vi "VI Tree - dictionary__ogtk.vi"   [LabVIEW 2018]
uses:
  <userlib>/_OpenG.lib/dictionary/dictionary.llb/Dictionary Key Value Pair Cluster__ogtk.ctl
panel:
  # "Dictionary VI Tree"
  # "Dictionary - VI Tree\n\nA VI that contains all of the Dictionary VIs\n\nPlease visit http://www.OpenG.org to learn about the\nOpen Source LabVIEW software movement.\n\nNOTICE -- YOU MUST LEAVE THIS NOTICE IN PLACE.  PER THE TERMS OF THE LICENSE BELOW, YOU MAY SUBLICENSE THIS SOFTWARE \nIN ANY WAY THAT DOES NOT CONFLICT WITH THIS LICENSE.\n\n### BSD License (http://www.opensource.org/licenses/bsd-license.php) Begin ###\n \nCopyright (c) 2005, Jim Kring <jim@jimkring.com>\n\nAll rights reserved.\n\nRedistribution and use in source and binary forms, with or without modification, are permitted provided that the following conditions are met:\n\n    * Redistributions of source code must retain the above copyright notice, this list of conditions and the following disclaimer.\n    * Redistributions in binary form must reproduce the above copyright notice, this list of conditions and the following disclaimer in the \n       documentation and/or other materials provided with the distribution.\n    * Neither the name of SciWare, James Kring, Inc., nor the names of its contributors may be used to endorse or promote products derived \n       from this software without specific prior written permission.\n\nTHIS SOFTWARE IS PROVIDED BY THE COPYRIGHT HOLDERS AND CONTRIBUTORS \"AS IS\" AND ANY EXPRESS OR IMPLIED WARRANTIES, \nINCLUDING, BUT NOT LIMITED TO, THE IMPLIED WARRANTIES OF MERCHANTABILITY AND FITNESS FOR A PARTICULAR PURPOSE ARE \nDISCLAIMED. IN NO EVENT SHALL THE COPYRIGHT OWNER OR CONTRIBUTORS BE LIABLE FOR ANY DIRECT, INDIRECT, INCIDENTAL,\n SPECIAL, EXEMPLARY, OR CONSEQUENTIAL DAMAGES (INCLUDING, BUT NOT LIMITED TO, PROCUREMENT OF SUBSTITUTE GOODS OR \nSERVICES; LOSS OF USE, DATA, OR PROFITS; OR BUSINESS INTERRUPTION) HOWEVER CAUSED AND ON ANY THEORY OF LIABILITY, \nWHETHER IN CONTRACT, STRICT LIABILITY, OR TORT (INCLUDING NEGLIGENCE OR OTHERWISE) ARISING IN ANY WAY OUT OF THE USE \nOF THIS SOFTWARE, EVEN IF ADVISED OF THE POSSIBILITY OF SUCH DAMAGE.\n\n### BSD License End ###"
types:
  T1 = typedef "Dictionary Key Value Pair Cluster__ogtk.ctl" = cluster{"key":variant, "value":variant}
  T2 = typedef "Dictionary Object RefNum__ogtk.ctl" = refnum<k1>
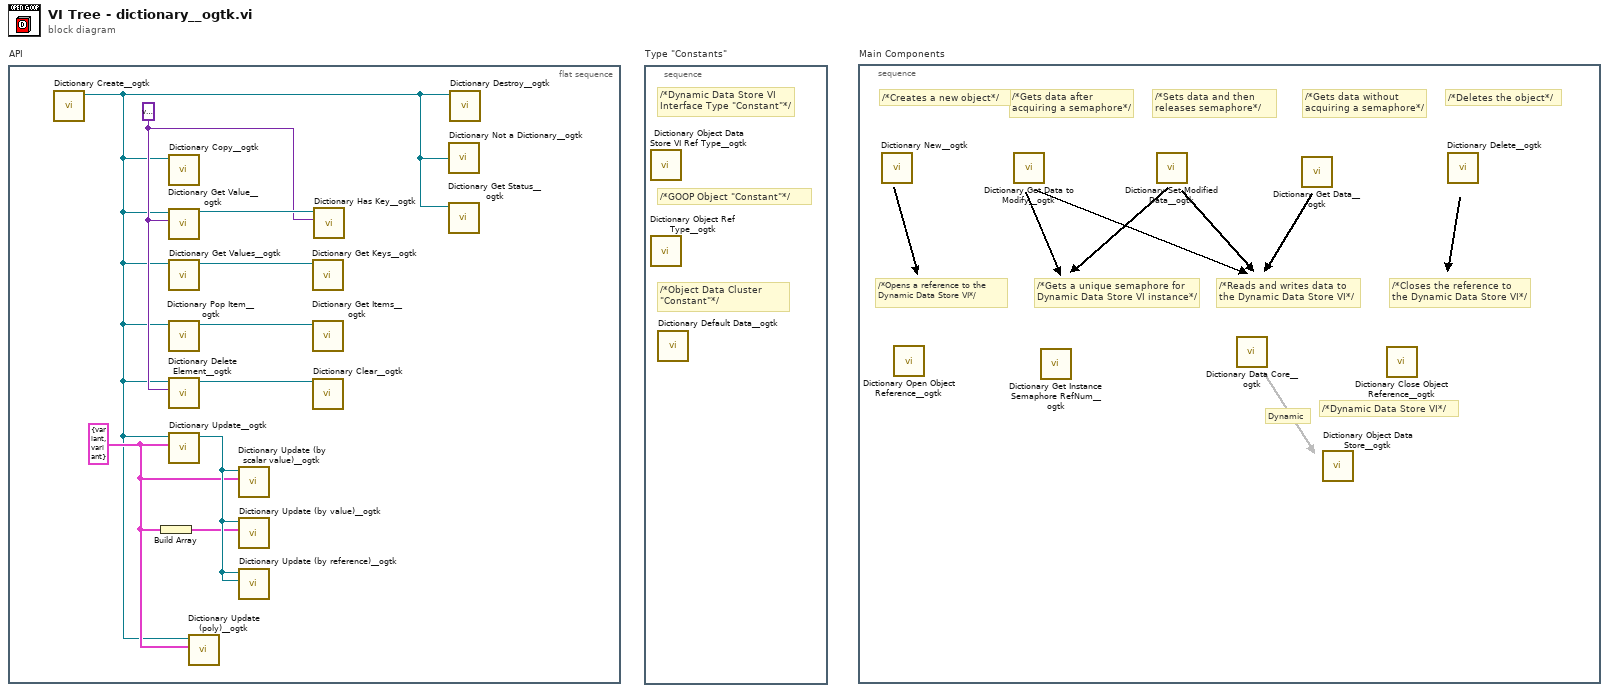
[diagram p0: block diagram]
diagram:
  n1 = flat-sequence "API" {
    frame #0 {
      w2 = T1 {"key"=variant, "value"=variant} ("key-value")
      w3 = variant ("key")
      n2 = call <userlib>:"Dictionary Create__ogtk.vi"() -> ("dictionary out"=w1:T2)  [unwired: 10 in, 1 out]
      n3 = Build Array(w2) -> (w4:T1[])
      n4 = call <userlib>:"Dictionary Copy__ogtk.vi"("dictionary"=w1) -> ()  [unwired: 8 in, 3 out]
      n5 = call <userlib>:"Dictionary Get Value__ogtk.vi"("key"=w3, "dictionary"=w1) -> ("dictionary out"=w5:T2)  [unwired: 6 in, 3 out]
      n6 = call <userlib>:"Dictionary Get Values__ogtk.vi"("dictionary"=w1) -> ("dictionary out"=w9:T2)  [unwired: 8 in, 2 out]
      n7 = call <userlib>:"Dictionary Pop Item__ogtk.vi"("dictionary"=w1) -> ("dictionary out"=w7:T2)  [unwired: 8 in, 2 out]
      n8 = call <userlib>:"Dictionary Delete Element__ogtk.vi"("key"=w3, "dictionary"=w1) -> ("dictionary out"=w6:T2)  [unwired: 8 in, 1 out]
      n9 = call-poly <userlib>:"Dictionary Update__ogtk.vi"("key-value"=w2, "dictionary"=w1) -> ("dictionary out"=w8:T2)  [unwired: 7 in, 2 out]
      n10 = call-poly <userlib>:"Dictionary Update (poly)__ogtk.vi"("key-value"=w2, "dictionary"=w1) -> ()  [unwired: 7 in, 3 out]
      n11 = call <userlib>:"Dictionary Update (by scalar value)__ogtk.vi"("key-value"=w2, "dictionary"=w8) -> ()  [unwired: 7 in, 3 out]
      n12 = call <userlib>:"Dictionary Update (by value)__ogtk.vi"("dictionary with updates"=w4, "dictionary"=w8) -> ()  [unwired: 7 in, 3 out]
      n13 = call <userlib>:"Dictionary Update (by reference)__ogtk.vi"("dictionary with updates"=w8, "dictionary"=w8) -> ()  [unwired: 7 in, 3 out]
      n14 = call <userlib>:"Dictionary Get Keys__ogtk.vi"("dictionary"=w9) -> ()  [unwired: 8 in, 3 out]
      n15 = call <userlib>:"Dictionary Get Items__ogtk.vi"("dictionary"=w7) -> ()  [unwired: 8 in, 3 out]
      n16 = call <userlib>:"Dictionary Clear__ogtk.vi"("dictionary"=w6) -> ()  [unwired: 9 in, 2 out]
      n17 = call <userlib>:"Dictionary Has Key__ogtk.vi"("key"=w3, "dictionary"=w5) -> ()  [unwired: 7 in, 3 out]
      n18 = call <userlib>:"Dictionary Not a Dictionary__ogtk.vi"("dictionary"=w1) -> ()  [unwired: 1 out]
      n19 = call <userlib>:"Dictionary Get Status__ogtk.vi"("dictionary"=w1) -> ()  [unwired: 8 in, 3 out]
      n20 = call <userlib>:"Dictionary Destroy__ogtk.vi"("dictionary"=w1) -> ()  [unwired: 10 in, 1 out]
    }
  }
  n21 = stacked-sequence "Type \"Constants\"" {
    frame #0 {
      # "/*Dynamic Data Store VI Interface Type \"Constant\"*/"
      # "/*GOOP Object \"Constant\"*/"
      # "/*Object Data Cluster \"Constant\"*/"
      n22 = call <userlib>:"Dictionary Object Data Store VI Ref Type__ogtk.vi"() -> ()  [unwired: 5 in, 1 out]
      n23 = call <userlib>:"Dictionary Object Ref Type__ogtk.vi"() -> ()  [unwired: 5 in, 1 out]
      n24 = call <userlib>:"Dictionary Default Data__ogtk.vi"() -> ()  [unwired: 1 out]
    }
  }
  n25 = stacked-sequence "Main Components" {
    frame #0 {
      # "Dynamic"
      # "/*Opens a reference to the Dynamic Data Store VI*/"
      # "/*Reads and writes data to the Dynamic Data Store VI*/"
      # "/*Closes the reference to the Dynamic Data Store VI*/"
      # "/*Dynamic Data Store VI*/"
      # "/*Gets a unique semaphore for Dynamic Data Store VI instance*/"
      # "/*Creates a new object*/"
      # "/*Gets data after acquiring a semaphore*/"
      # "/*Sets data and then releases semaphore*/"
      # "/*Deletes the object*/"
      # "/*Gets data without acquiring a semaphore*/"
      n26 = call <userlib>:"Dictionary New__ogtk.vi"() -> ()  [unwired: 10 in, 2 out]
      n27 = call <userlib>:"Dictionary Open Object Reference__ogtk.vi"() -> ()  [unwired: 10 in, 2 out]
      n28 = call <userlib>:"Dictionary Get Data to Modify__ogtk.vi"() -> ()  [unwired: 8 in, 4 out]
      n29 = call <userlib>:"Dictionary Get Instance Semaphore RefNum__ogtk.vi"() -> ()  [unwired: 9 in, 3 out]
      n30 = call <userlib>:"Dictionary Set Modified Data__ogtk.vi"() -> ()  [unwired: 10 in, 2 out]
      n31 = call <userlib>:"Dictionary Data Core__ogtk.vi"() -> ()  [unwired: 9 in, 3 out]
      n32 = call <userlib>:"Dictionary Get Data__ogtk.vi"() -> ()  [unwired: 9 in, 3 out]
      n33 = call <userlib>:"Dictionary Object Data Store__ogtk.vi"() -> ()  [unwired: 11 in, 1 out]
      n34 = call <userlib>:"Dictionary Close Object Reference__ogtk.vi"() -> ()  [unwired: 11 in, 1 out]
      n35 = call <userlib>:"Dictionary Delete__ogtk.vi"() -> ()  [unwired: 11 in, 1 out]
    }
  }
